vi "FGV DAB.vi"(10 "HR/SC":dbl[][](array[numeric]), 11 "Enum":T1) -> (3 "DAB":dbl[][](array[numeric]))   [LabVIEW 2014]
uses:
  set_get.ctl
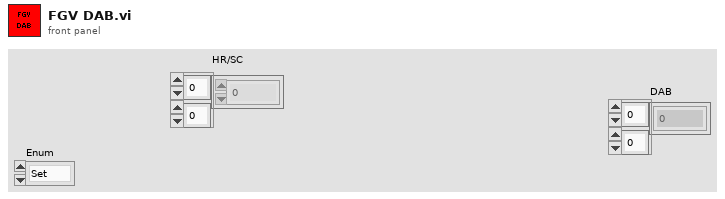
[diagram p1: front panel]
types:
  T1 = typedef "set_get.ctl" = enum16{"Set", "Get"}
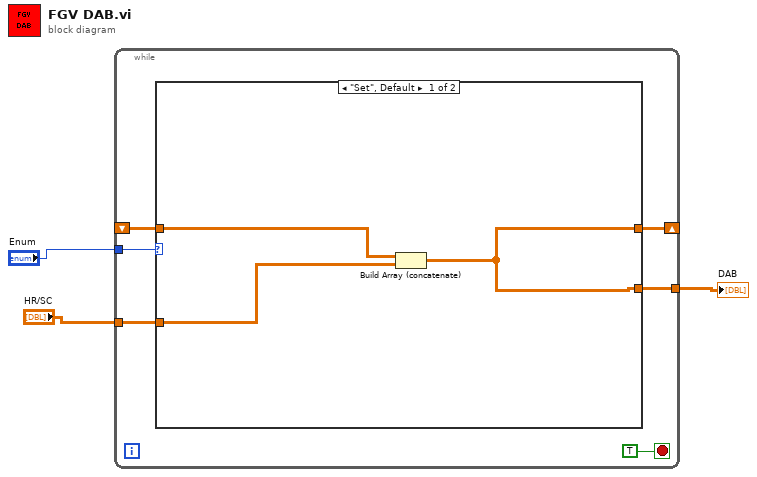
[diagram p0: block diagram]
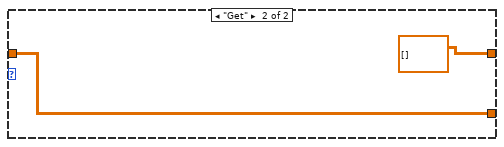
[diagram p2: hidden frame]
diagram:
  n1 = while {
    tunnel: "Enum" -> [w9]
    tunnel: "HR/SC" -> [w8]
    shift-right: [w7] -> _
    shift-left: _ -> [w6]
    tunnel: [w4] -> w1
    stop <- TRUE stop-if-true
    n2 = case shown="\"Set\", Default" w9 {
      tunnel: w8 -> [w11 _]
      tunnel: [w10 dbl[][] []] -> w7
      tunnel: w6 -> [w12 w14]
      tunnel: [w10 w14] -> w4
      frame "Set", Default {
        n3 = Build Array (concatenate)(w12, w11) -> (w10:dbl[][])
      }
      frame "Get" {
      }
    }
  }
  "DAB" <- w1
